vi "PCSMain.Free PHELIX Motion Instances.vi"(1 "DB Entries":cluster{"Object Name":string, "Class":string}[](array[cluster])) -> (0 "Free Motion GUI elements":cluster{"Object Name":string, "Class":string}[](array[cluster]))   [LabVIEW 2014, in "PCSMain.lvlib"]
doc: "This VI acts as a filter: From the input data base entries, it gives out all entries which are belonging to the classes NF_AxisGUI_NF, PH_AxisGUI_NF2, PH_AxisGUI_6P, PH_4_pos_Selector, and PH_Waveplate-GUI_6P except those named in the listboxes - those are also kicked out. Inside the block diagram may be others are kicked out which are inserted by hand. This VI is meant to be used in MainGUIs."
uses:
  PCSMain.lvlib
  PH_Beamline/PH_Beamline.Motion GUI Instances.ctl
  PH_Beamline/PH_Beamline.Switch+6P Instances.ctl
  Z6_Beamline/Z6_Beamline.Motion GUI Instances.ctl
  Z6_Beamline/Z6_Beamline.Switch+6P Instances.ctl
  PH_Beamline/PH_Beamline.6P 4 Pos Selector Instances.ctl
  PH_Beamline/PH_Beamline.6P Revolver GUI Instances.ctl
  PH_Beamline/PH_Beamline.lvlib
  Z6_Beamline/Z6_Beamline.lvlib
panel:
  in  "6P Revolver GUI Instances":T1="MAS_Discrete_Spectro_Rev6PGUI"
  in  "6P 4 Pos Selector Instances":T2="PA_MA_T3_Exit_6P4QGUI"
  in  "Z6 Switch and 6P Instances":T3="N/A"
  in  "Z6 Motion GUI Instances":T4="Z6_MM10_6PGUI"
  in  "Switch and 6P Instances":T5="BL_Position_MM5::MA_MM5_6PGUI"
  in  "Motion GUI Instances":T6="MA_MM1_AxisGUI"
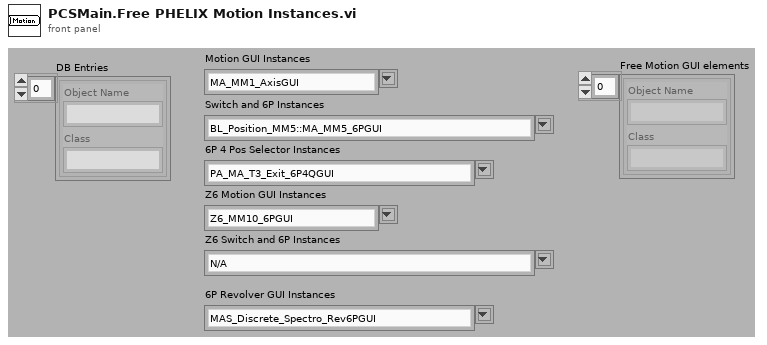
[diagram p1: front panel]
types:
  T1 = typedef "PH_Beamline.lvlib/PH_Beamline.6P Revolver GUI Instances.ctl" = string
  T2 = typedef "PH_Beamline.lvlib/PH_Beamline.6P 4 Pos Selector Instances.ctl" = string
  T3 = typedef "Z6_Beamline.lvlib/Z6_Beamline.Switch+6P Instances.ctl" = string
  T4 = typedef "Z6_Beamline.lvlib/Z6_Beamline.Motion GUI Instances.ctl" = string
  T5 = typedef "PH_Beamline.lvlib/PH_Beamline.Switch+6P Instances.ctl" = string
  T6 = typedef "PH_Beamline.lvlib/PH_Beamline.Motion GUI Instances.ctl" = string
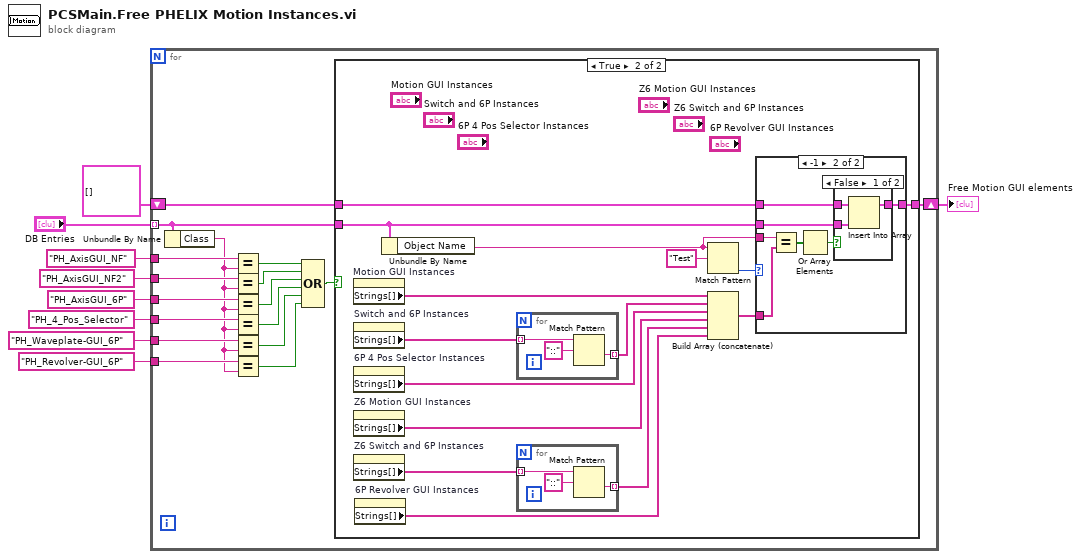
[diagram p0: block diagram]
diagram:
  n1 = for {
    tunnel: "DB Entries" -> [w26] mode=indexing
    shift-right: [w25] -> w9
    shift-left: cluster{"Object Name":string, "Class":string}[] [] -> [w24]
    tunnel: "PH_AxisGUI_NF" ("Class") -> [w15]
    tunnel: "PH_AxisGUI_6P" ("Class") -> [w18]
    tunnel: "PH_AxisGUI_NF2" ("Class") -> [w20]
    tunnel: "PH_4_Pos_Selector" ("Class") -> [w16]
    tunnel: "PH_Waveplate-GUI_6P" ("Class") -> [w14]
    tunnel: "PH_Revolver-GUI_6P" -> [w11]
    n2 = Unbundle By Name(w26) -> ("Class"=w10:string)
    n3 = Equal?(x=w15, y=w10) -> (x = y?=w22:bool)
    n4 = Equal?(x=w20, y=w10) -> (x = y?=w19:bool)
    n5 = Equal?(x=w18, y=w10) -> (x = y?=w21:bool)
    n6 = Equal?(x=w16, y=w10) -> (x = y?=w17:bool)
    n7 = Equal?(x=w14, y=w10) -> (x = y?=w13:bool)
    n8 = Equal?(x=w11, y=w10) -> (x = y?=w12:bool)
    n9 = Compound Arithmetic op=OR(w22, w19, w21, w17, w13, w12) -> (w23:bool)
    n10 = case shown="True" w23 {
      tunnel: w26 -> [_ w40]
      tunnel: [w27 w42] -> w25
      tunnel: w24 -> [w27 w41]
      frame False {
      }
      frame True {
        n11 = property on="Motion GUI Instances" class="CmbBox (strict)"() -> ("Strings[]"=w33:string[])  [unwired: 2 in, 2 out]
        n12 = property on="Switch and 6P Instances" class="CmbBox (strict)"() -> ("Strings[]"=w32:string[])  [unwired: 2 in, 2 out]
        n13 = property on="6P 4 Pos Selector Instances" class="CmbBox (strict)"() -> ("Strings[]"=w29:string[])  [unwired: 2 in, 2 out]
        n14 = property on="Z6 Motion GUI Instances" class="CmbBox (strict)"() -> ("Strings[]"=w31:string[])  [unwired: 2 in, 2 out]
        n15 = property on="Z6 Switch and 6P Instances" class="CmbBox (strict)"() -> ("Strings[]"=w30:string[])  [unwired: 2 in, 2 out]
        n16 = property on="6P Revolver GUI Instances" class="CmbBox (strict)"() -> ("Strings[]"=w28:string[])  [unwired: 2 in, 2 out]
        n17 = Unbundle By Name(w40) -> ("Object Name"=w37:string)
        n18 = for {
          tunnel: w32 -> [w48] mode=indexing
          tunnel: [w46] -> w35 mode=indexing
          n19 = Match Pattern(string=w48, regular expression="::") -> (after substring=w46:string)  [unwired: 1 in, 3 out]
        }
        n20 = for {
          tunnel: w30 -> [w45] mode=indexing
          tunnel: [w43] -> w34 mode=indexing
          n21 = Match Pattern(string=w45, regular expression="::") -> (after substring=w43:string)  [unwired: 1 in, 3 out]
        }
        n22 = Match Pattern(string=w37, regular expression="Test") -> (offset past match=w38:i32)  [unwired: 1 in, 3 out]
        n23 = Build Array (concatenate)(w33, w35, w29, w31, w34, w28) -> (w36:string[])
        n24 = case shown="-1" w38 {
          tunnel: [w49 w56] -> w42
          tunnel: w41 -> [w49 w55]
          tunnel: w40 -> [_ w54]
          tunnel: w37 -> [_ w53]
          tunnel: w36 -> [_ w52]
          frame 0, Default {
          }
          frame -1 {
            n25 = Equal?(x=w53, y=w52) -> (x = y?=w51:bool[])
            n26 = Or Array Elements(Boolean array=w51) -> (logical OR=w50:bool)
            n27 = case shown="False" w50 {
              tunnel: [w59 w60] -> w56
              tunnel: w55 -> [w58 w60]
              tunnel: w54 -> [w57 _]
              frame False {
                n28 = Insert Into Array(array=w58, new element=w57) -> (w59:cluster{"Object Name":string, "Class":string}[])  [unwired: 1 in]
              }
              frame True {
              }
            }
          }
        }
      }
    }
  }
  "Free Motion GUI elements" <- w9
